vi "Test Response.vi"() -> ()   [LabVIEW 2020]
doc: "Use this template to build a producer/consumer design pattern with events to produce queue items. Use this design pattern instead of the User Interface Event Handler pattern for user interfaces when you want to execute code asynchronously in response to an event without slowing the user interface responsiveness."
uses:
  Labview Library/Libraries/HW_NI_CTR/NI DAQ Counter/NI DAQ Counter.lvlib
  Labview Library/Libraries/Basic Experiment/Basic Experiment.lvlib
  Labview Library/Libraries/Basic Experiment/1AutoTrace Settings.ctl
panel:
  out "Final Position":dbl
  in  "Single axis Settings":T1={"Axis"=enum."z", "Sample Rate (Hz)"=20.0, "Diameter(um)"=6.0, "Num"=25, "Peak Threshold"=4500.0, "First Wait(ms)"=20, "Move wait(ms)"=20, "Final Wait(ms)"=30, "Read Final"=FALSE} {"Num" format="%#_13g"}
  in  "Move Step":dbl=1.0 format="%#_13g"
  in  "milliseconds to wait":u32
  in  "Numeric":i32=250
  out "Z轴位移响应速度测试":dbl[](graph)
  in  "Enqueue Element":bool
  in  "stop":bool
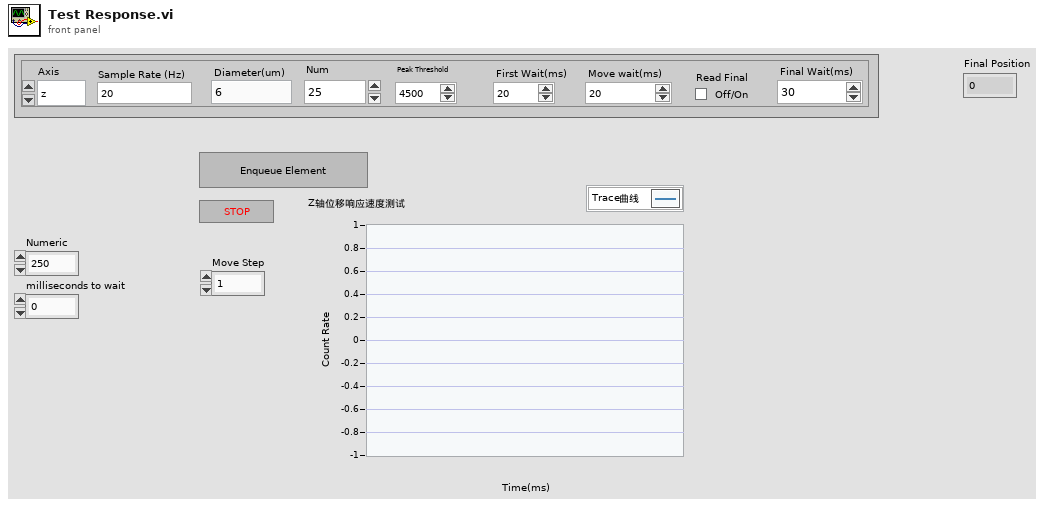
[diagram p1: front panel]
types:
  T1 = typedef "Basic Experiment.lvlib/1AutoTrace Settings.ctl" = cluster{"Axis":enum16{"x", "y", "z"}, "Sample Rate (Hz)":dbl, "Diameter(um)":dbl, "Num":i32, "Peak Threshold":dbl, "First Wait(ms)":u32, "Move wait(ms)":u32, "Final Wait(ms)":u32, "Read Final":bool}
  T2 = enum16{"Config Mode", "Slow Mode", "Test Mode", "Default Mode"}
  T3 = typedef "Basic Experiment.lvlib/1AutoTrace Results.ctl" = cluster{"Start Point":dbl, "Peak Position":dbl, "Final Count":dbl, "Peak Count":dbl, "Axis":enum16{"X", "Y", "Z"}, "Raw Tdms Path":path, "Raw Image Path":path, "Final Position":dbl, "Background":dbl}
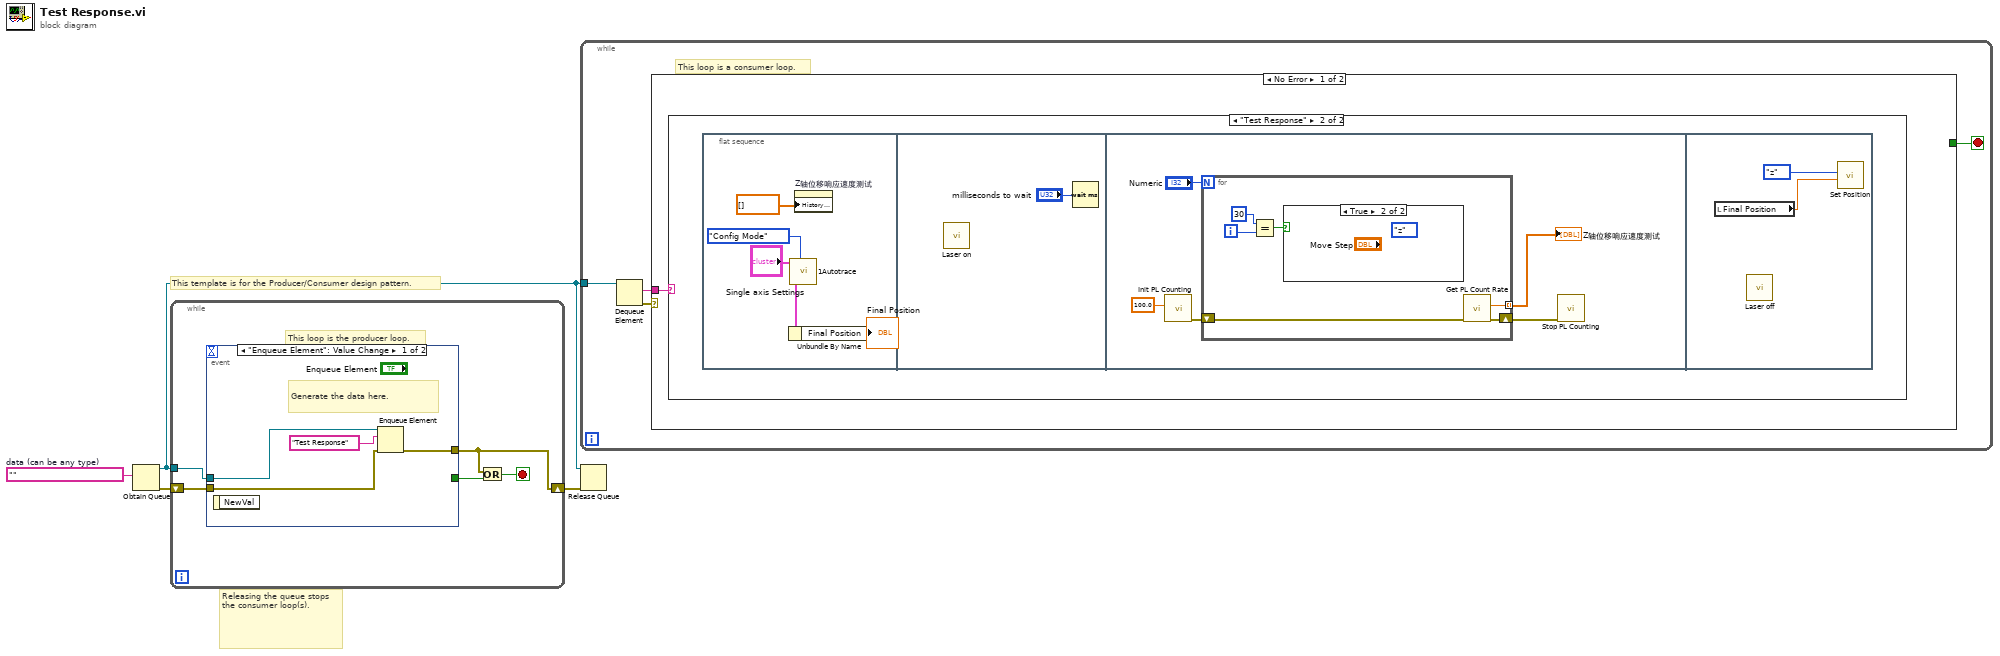
[diagram p0: block diagram]
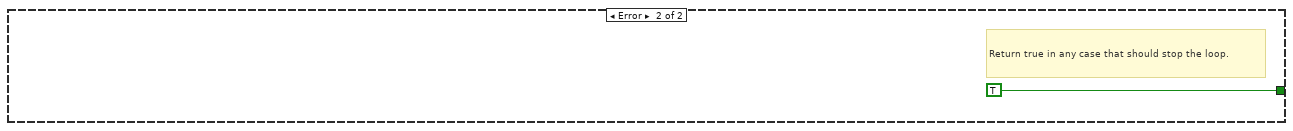
[diagram p4: hidden frame]
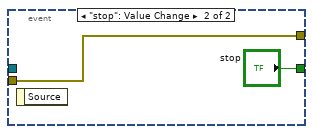
[diagram p5: hidden frame]
diagram:
  w2 = ""  # data (can be any type)
  # "Releasing the queue stops the consumer loop(s)."
  # "This template is for the Producer/Consumer design pattern."
  n1 = Obtain Queue(element data type=w2) -> (queue out=w1:refnum<queue>, error out=w4:errorcluster)  [unwired: 4 in, 1 out]
  n2 = while {
    shift-right: [w5] -> w3
    shift-left: w4 -> [w8]
    tunnel: w1 -> [w9]
    stop <- w6 stop-if-true
    # "This loop is the producer loop."
    n3 = event shown="[0] \"Enqueue Element\": Value Change" {
      selector: _ -> [_ _]
      dyn-events: _ -> [_ _]
      timeout: _ -> [_ _]
      tunnel: w9 -> [w13 _]
      tunnel: w8 -> [w12 w14]
      tunnel: [w11 w14] -> w5
      tunnel: [_ "stop"] -> w7
      event "Enqueue Element": Value Change {
        # "Generate the data here."
        n4 = event-data() -> ()  [unwired: 1 in, 1 out]
        n5 = Enqueue Element(queue=w13, element="Test Response", error in (no error)=w12) -> (error out=w11:errorcluster)  [unwired: 1 in, 2 out]
      }
      event "stop": Value Change {
        n6 = event-data() -> ()  [unwired: 1 in, 1 out]
      }
    }
    n7 = Or(x=w5, y=w7) -> (x .or. y?=w6:bool)
  }
  n8 = while {
    tunnel: w1 -> [w19]
    stop <- w16 stop-if-true
    # "This loop is a consumer loop."
    n9 = Dequeue Element(queue=w19) -> (element=w17:string, error out=w18:errorcluster)  [unwired: 2 in, 2 out]
    n10 = case shown="No Error" w18 {
      tunnel: w17 -> [w20 _]
      tunnel: [_ TRUE] -> w16
      frame No Error {
        n11 = case shown="\"Test Response\"" w20 {
          frame "False", Default {
          }
          frame "Test Response" {
            n12 = flat-sequence {
              frame #0 {
                n13 = call "1Autotrace.vi"("Mode"=T2."Config Mode", "Single axis Settings"="Single axis Settings") -> ("Single AutoTrace Result"=w22:T3)  [unwired: 7 in, 2 out]
                n14 = Unbundle By Name(w22) -> ("Final Position"=→"Final Position":dbl)
                n15 = property on="Z轴位移响应速度测试" class="WFChart (strict)"("History Data"=dbl[] []) -> ()  [unwired: 2 in, 2 out]
              }
              frame #1 {
                n16 = call "Laser on.vi"() -> ()  [unwired: 11 in, 1 out]
                n17 = Wait (ms)(milliseconds to wait="milliseconds to wait") -> ()  [unwired: 1 out]
              }
              frame #2 {
                n18 = call "Init PL Counting.vi"("Sample Rate (Hz)"=100.0) -> ("error out"=w30:errorcluster)  [unwired: 10 in]
                n19 = for {
                  N: "Numeric" -> [_]
                  shift-right: [w36] -> w29
                  shift-left: w30 -> [w37]
                  tunnel: [w35] -> w27 mode=indexing
                  i -> [w34]
                  n20 = Equal?(x=30, y=w34) -> (x = y?=w32:bool)
                  n21 = case shown="True" w32 {
                    frame False {
                    }
                    frame True {
                      (unwired) enum16{"x", "y", "z"}."z" ("Axis To Move")
                    }
                  }
                  n22 = call "Get PL Count Rate.vi"("error in"=w37) -> ("error out"=w36:errorcluster, "Count Rate"=w35:dbl)  [unwired: 9 in]
                }
                "Z轴位移响应速度测试" <- w27
                n23 = call "Stop PL Counting.vi"("error in"=w29) -> ()  [unwired: 10 in, 1 out]
              }
              frame #3 {
                n24 = local read "Final Position"() -> (w39:dbl)
                n25 = call "Laser off.vi"() -> ()  [unwired: 11 in, 1 out]
                n26 = call "Set Position.vi"(9:w39, "Position"=enum16{"x", "y", "z"}."z" ("Axis To Move")) -> ()  [unwired: 9 in, 1 out]
              }
            }
          }
        }
      }
      frame Error {
        # "Return true in any case that should stop the loop."
      }
    }
  }
  n27 = Release Queue(queue=w1, error in (no error)=w3) -> ()  [unwired: 1 in, 3 out]
